vi "Open Motor.vi"(0 "Control Mode":T5, 1 "PID?":bool, 2 "Feedback Reference":T6, 4 "error in":errorcluster, 5 "refnum name":string="My Motor RefNum", 7 "mode (safety config)":T8, 9 "CAN Device Number":u8, 11 "Set sensor position":dbl, 12 "Reverse Feedback Sensor":bool, 13 "PID gains":T7={"proportional gain (Kc)"=5.0, "integral time (Ti, min)"=0.032, "derivative time (Td, min)"=0.0} {"derivative time (Td, min)" format="%.3f"; "integral time (Ti, min)" format="%.8f"; "proportional gain (Kc)" format="%.8f"}) -> (6 "CAN Talon SRX Ref":T1={"DeviceStatus"={"status"=FALSE, "code"=0, "source"=""}, "Type"=enum."PWM", "PWM"={"PWM Channel"=enum."PWM 1", "DeadBand"={"Name"="", "maxPositivePwm"=0, "minPositivePwm"=0, "centerPwm"=0, "maxNegativePwm"=0, "minNegativePwm"=0, "angularRange"=0}}, "CAN"={"Device Number"=0, "SetOutput VI Ref"=variant(enum8{"Percent VBus", "Current", "Speed", "Position", "Voltage"} enum."Percent VBus"), "GetOutput VI Ref"=variant(refnum<k1> refnum), "Enable VI Ref"=variant(dbl 12.0), "Disable VI Ref"=variant(enum8{"Percent VBus", "Speed", "Position", "Slave", "Unchanged / Invalid", "Voltage Compensation", "Current", "Motion Profile"} enum."Percent VBus"), "Data"=variant}, "Invert"=FALSE}, 15 "error out":errorcluster)   [LabVIEW 2016, in "Huskie Swerve.lvlib"]
uses:
  Huskie Swerve.lvlib
  <vilib>/Rock Robotics/WPI/SafetyOutput/WPI_SafetyOutputConfigMenu.ctl
  <vilib>/Rock Robotics/WPI/ThirdParty/CanMotor/TalonSRX/WPI_CANTalonSRX_APIFeedbackSelect.ctl
  <vilib>/Rock Robotics/WPI/ThirdParty/CanMotor/TalonSRX/WPI_CANTalonSRX_APIControlMode.ctl
  <vilib>/Rock Robotics/WPI/MotorControl/WPI_MotorControlDeviceRef.ctl
  <vilib>/Rock Robotics/WPI/MotorControl/WPI_MotorControlType.ctl
  <vilib>/Rock Robotics/SystemInterfaces/DIO/FPGA_DIOPWMChannel.ctl
  <vilib>/Rock Robotics/WPI/PWM/WPI_PWMDeadband.ctl
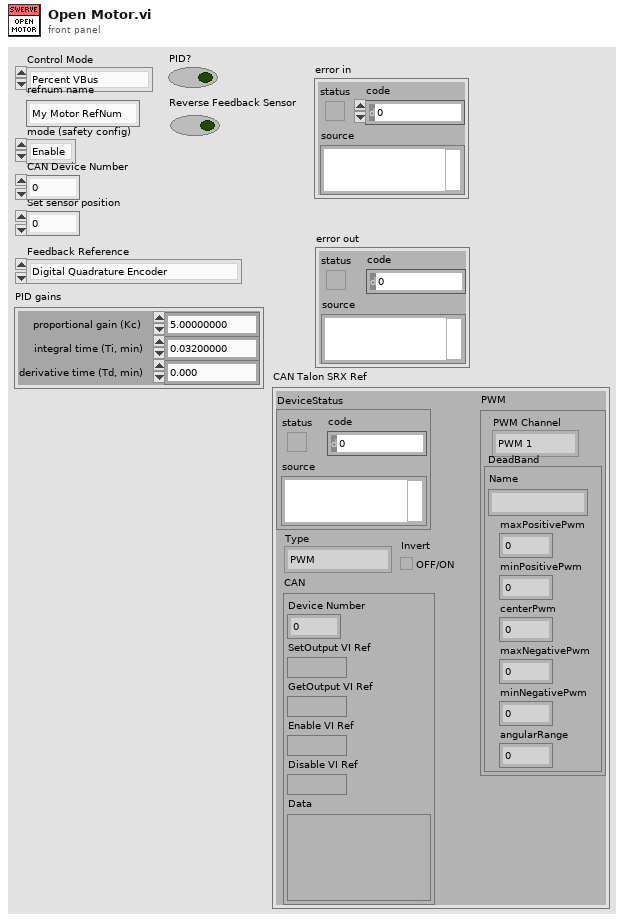
[diagram p1: front panel]
types:
  T1 = typedef "WPI_MotorControlDeviceRef.ctl" = cluster{"DeviceStatus":errorcluster, "Type":T2, "PWM":cluster{"PWM Channel":T3, "DeadBand":T4}, "CAN":cluster{"Device Number":u8, "SetOutput VI Ref":variant, "GetOutput VI Ref":variant, "Enable VI Ref":variant, "Disable VI Ref":variant, "Data":variant}, "Invert":bool}
  T2 = typedef "WPI_MotorControlType.ctl" = enum16{"PWM", "CAN"}
  T3 = typedef "FPGA_DIOPWMChannel.ctl" = enum8{"PWM 0", "PWM 1", "PWM 2", "PWM 3", "PWM 4", "PWM 5", "PWM 6", "PWM 7", "PWM 8", "PWM 9", "PWM MXP 0", "PWM MXP 1", "PWM MXP 2", "PWM MXP 3", "PWM MXP 4", "PWM MXP 5", "PWM MXP 6", "PWM MXP 7", "PWM MXP 8", "PWM MXP 9", "Invalid"}
  T4 = typedef "WPI_PWMDeadband.ctl" = cluster{"Name":string, "maxPositivePwm":i32, "minPositivePwm":i32, "centerPwm":i32, "maxNegativePwm":i32, "minNegativePwm":i32, "angularRange":u16}
  T5 = typedef "WPI_CANTalonSRX_APIControlMode.ctl" = enum8{"Percent VBus", "Speed", "Position", "Slave", "Unchanged / Invalid", "Voltage Compensation", "Current", "Motion Profile", "Motion Magic"}
  T6 = typedef "WPI_CANTalonSRX_APIFeedbackSelect.ctl" = enum16{"Digital Quadrature Encoder", "Analog Potentiometer", "Analog Encoder", "Count on Quad-A (Rising-Edge)", "Count on Quad-A (Falling-Edge)", "CTR Magnetic Enc (Absolute)", "CTR Magnetic Enc (Relative)", "Pulse Width"}
  T7 = cluster{"proportional gain (Kc)":dbl, "integral time (Ti, min)":dbl, "derivative time (Td, min)":dbl}
  T8 = typedef "WPI_SafetyOutputConfigMenu.ctl" = enum16{"Enable", "Disable"}
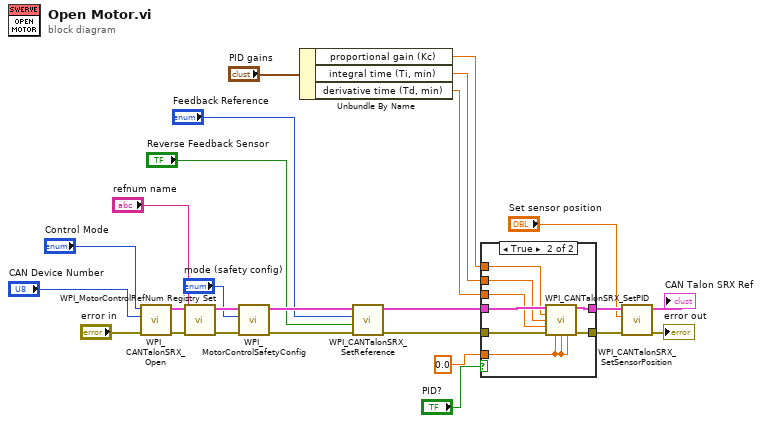
[diagram p0: block diagram]
diagram:
  n1 = call <vilib>:"WPI_CANTalonSRX_Open.vi"("error in"="error in", "Device Number"="CAN Device Number", "Control Mode"="Control Mode") -> ("error out"=w25:errorcluster, "CAN Talon SRX Ref"=w26:T1)  [unwired: 7 in]
  n2 = call <vilib>:"WPI_MotorControlRefNum Registry Set.vi"("error in (no error)"=w25, "refnum name"="refnum name", "MotorControlDevRef"=w26) -> ("error out"=w20:errorcluster, "MotorControlDevRef"=w23:T1)  [unwired: 7 in]
  n3 = call <vilib>:"WPI_MotorControlSafetyConfig.vi"("error in (no error)"=w20, "mode"="mode (safety config)", "MotorControlDevRef"=w23) -> ("error out"=w21:errorcluster, "MotorControlDevRef"=w22:T1)  [unwired: 7 in]
  n4 = Unbundle By Name("PID gains") -> ("proportional gain (Kc)"=w10:dbl, "integral time (Ti, min)"=w9:dbl, "derivative time (Td, min)"=w8:dbl)
  n5 = call <vilib>:"WPI_CANTalonSRX_SetReference.vi"("error in (no error)"=w21, "Reverse Feedback Sensor"="Reverse Feedback Sensor", "Feedback Reference"="Feedback Reference", "CAN Talon SRX Ref"=w22) -> ("error out"=w18:errorcluster, "CAN Talon SRX Ref"=w19:T1)  [unwired: 6 in]
  n6 = case shown="True" "PID?" {
    tunnel: w19 -> [w28 w36]
    tunnel: w18 -> [w27 w35]
    tunnel: [w27 w34] -> w17
    tunnel: [w28 w33] -> w16
    tunnel: w10 -> [_ w32]
    tunnel: w9 -> [_ w31]
    tunnel: w8 -> [_ w30]
    tunnel: 0.0 ("New Sensor Position") -> [_ w29]
    frame False {
    }
    frame True {
      n7 = call <vilib>:"WPI_CANTalonSRX_SetPID.vi"("CAN Talon SRX Ref"=w36, "P"=w32, "I"=w31, "D"=w30, "error in (no error)"=w35, "F"=w29, "I Zone"=w29, "Ramp Rate"=w29) -> ("CAN Talon SRX Ref"=w33:T1, "error out"=w34:errorcluster)  [unwired: 6 in]
    }
  }
  n8 = call <vilib>:"WPI_CANTalonSRX_SetSensorPosition.vi"("error in (no error)"=w17, "New Sensor Position"="Set sensor position", "CAN Talon SRX Ref"=w16) -> ("error out"=→"error out":errorcluster, "CAN Talon SRX Ref"=→"CAN Talon SRX Ref":T1)  [unwired: 7 in]
